vi "io_write_with_OPC_synchro.vi"(4 "Send *ESR? at the end (T)":bool=TRUE, 7 "Timeout in (0 = OPC timeout)":u32, 8 "error in":errorcluster, 10 "write buffer":string, 11 "VISA resource name":refnum<visa-resource-name>) -> (0 "error out":errorcluster, 3 "VISA resource name out":refnum<visa-resource-name>)   [LabVIEW 2014, in "rszvl_rsidr_core.lvlib"]
uses:
  rszvl_rsidr_core.lvlib
  type_Attribute.ctl
  type_Attribute_Data_Type.ctl
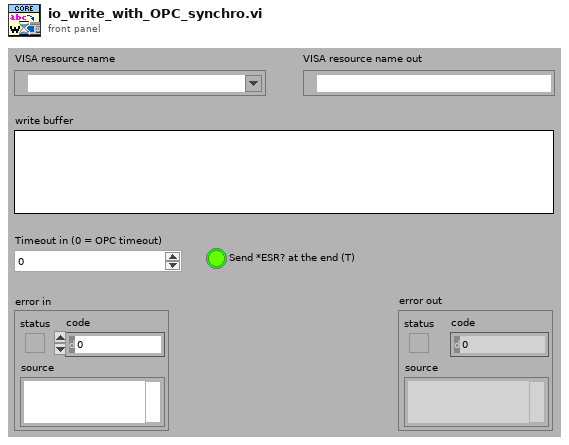
[diagram p1: front panel]
types:
  T1 = typedef "rszvl_rsidr_core.lvlib/type_Session_Data.ctl" = cluster{"Instr type":string, "Instr type for err. msg.":string, "Installed Options":string[], "OPC Timeout":i32, "Query Instrument Status":bool, "Check Range":bool, "Check Options":bool, "Add LF to Write":bool, "Simulate":bool, "Logging":bool, "Logging params":variant, "Interface Type":enum16{"Unknown", "GPIB", "VXI", "GPIB_VXI", "ASRL", "PXI", "TCPIP", "USB", "SOCKET"}, "Fast Sweep":i32, "AdditionalFlags":i32, "WaitBeforeWrite":i32, "WaitBeforeRead":i32, "BinDataChunkSize":i64}
  T2 = enum16{"Unknown", "GPIB", "VXI", "GPIB_VXI", "ASRL", "PXI", "TCPIP", "USB", "SOCKET"}
  T3 = typedef "rszvl_rsidr_core.lvlib/type_Attribute.ctl" = cluster{"Identifier":string, "Descriptive name":string, "Data Type":T4, "Command":string, "Access":u16, "Range Table":string, "Read Callback":string, "Write Callback":string, "Range Callback":string, "Check Callback":string, "Rngtable Callback":string, "Coerce Callback":string, "Supported Models":string, "Instrument Options":string, "Repeated Capabilities":string, "Check Status Callback":string, "Index":i32, "Flag: OPC Wait":bool, "Flag: Dont check status":bool, "Flag: Cache Only":bool}
  T4 = typedef "rszvl_rsidr_core.lvlib/type_Attribute_Data_Type.ctl" = enum16{"Integer 32", "Double", "String", "Boolean", "None", "Integer 64"}
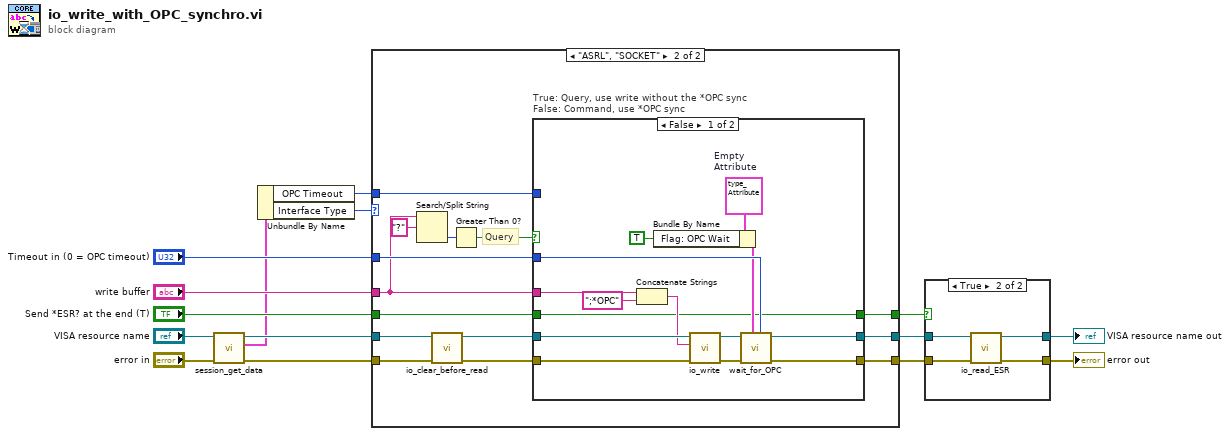
[diagram p0: block diagram]
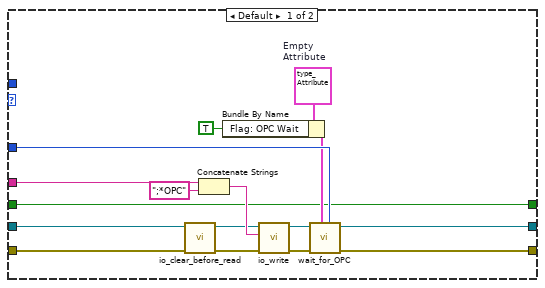
[diagram p3: hidden frame]
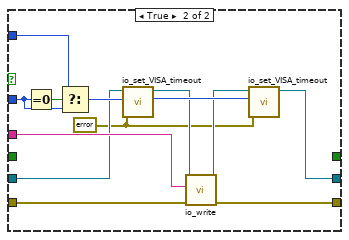
[diagram p4: hidden frame]
diagram:
  n1 = call "session_get_data.vi"("error in"="error in", "VISA resource name"="VISA resource name") -> ("error out"=w10:errorcluster, "Session User Data out"=w1:T1, "VISA resource name out"=w9:refnum<visa-resource-name>)  [unwired: 7 in]
  n2 = Unbundle By Name(w1) -> ("OPC Timeout"=w2:i32, "Interface Type"=w8:T2)
  n3 = case shown="\"ASRL\", \"SOCKET\"" w8 {
    tunnel: "Timeout in (0 = OPC timeout)" -> [w29 w45]
    tunnel: w10 -> [w28 w44]
    tunnel: w9 -> [w27 w43]
    tunnel: "write buffer" -> [w22 w37]
    tunnel: [w16 w36] -> w5
    tunnel: [w17 w35] -> w6
    tunnel: "Send *ESR? at the end (T)" -> [w18 w34]
    tunnel: [w18 w33] -> w7
    tunnel: w2 -> [_ w32]
    frame Default {
      w20 = T3 {"Identifier"="", "Descriptive name"="", "Data Type"=enum."Integer 32", "Command"="", "Access"=2, "Range Table"="", "Read Callback"="", "Write Callback"="", "Range Callback"="", "Check Callback"="", "Rngtable Callback"="", "Coerce Callback"="", "Supported Models"="", "Instrument Options"="", "Repeated Capabilities"="", "Check Status Callback"="", "Index"=0, "Flag: OPC Wait"=FALSE, "Flag: Dont check status"=FALSE, "Flag: Cache Only"=FALSE}  # Empty Attribute
      n4 = call "io_clear_before_read.vi"("error in"=w28, "VISA resource name"=w27) -> ("error out"=w26:errorcluster, "VISA resource name out"=w25:refnum<visa-resource-name>)  [unwired: 8 in]
      n5 = Concatenate Strings(w22, ";*OPC" ("string")) -> (w31:string)
      n6 = Bundle By Name(cluster=w20, "Flag: OPC Wait"=TRUE) -> (w19:T3)
      n7 = call "io_write.vi"("error in"=w26, "write buffer"=w31, "VISA resource name"=w25) -> ("error out"=w24:errorcluster, "VISA resource name out"=w23:refnum<visa-resource-name>)  [unwired: 7 in]
      n8 = call "wait_for_OPC.vi"("Timeout in (0 = OPC timeout)"=w29, "Attribute"=w19, "error in"=w24, "VISA resource name"=w23) -> ("error out"=w17:errorcluster, "VISA resource name out"=w16:refnum<visa-resource-name>)  [unwired: 6 in]
    }
    frame "ASRL", "SOCKET" {
      # "Query"
      n9 = Search/Split String(string=w37, search string/char (-)="?") -> (offset of match=w39:i32)  [unwired: 1 in, 2 out]
      n10 = call "io_clear_before_read.vi"("error in"=w44, "VISA resource name"=w43) -> ("error out"=w42:errorcluster, "VISA resource name out"=w41:refnum<visa-resource-name>)  [unwired: 8 in]
      n11 = Greater Than 0?(x=w39) -> (x > 0?=w38:bool)
      n12 = case "True: Query, use write without the *OPC sync\nFalse: Command, use *OPC sync" shown="False" w38 {
        tunnel: w37 -> [w51 w72]
        tunnel: w45 -> [w59 w70]
        tunnel: w42 -> [w58 w64]
        tunnel: w41 -> [w57 w67]
        tunnel: [w48 w62] -> w36
        tunnel: [w47 w63] -> w35
        tunnel: w34 -> [w46 _]
        tunnel: [w46 _] -> w33
        tunnel: w32 -> [_ w61]
        frame False {
          w53 = T3 {"Identifier"="", "Descriptive name"="", "Data Type"=enum."Integer 32", "Command"="", "Access"=2, "Range Table"="", "Read Callback"="", "Write Callback"="", "Range Callback"="", "Check Callback"="", "Rngtable Callback"="", "Coerce Callback"="", "Supported Models"="", "Instrument Options"="", "Repeated Capabilities"="", "Check Status Callback"="", "Index"=0, "Flag: OPC Wait"=FALSE, "Flag: Dont check status"=FALSE, "Flag: Cache Only"=FALSE}  # Empty Attribute
          n13 = Concatenate Strings(w51, ";*OPC" ("string")) -> (w49:string)
          n14 = Bundle By Name(cluster=w53, "Flag: OPC Wait"=TRUE) -> (w52:T3)
          n15 = call "io_write.vi"("error in"=w58, "write buffer"=w49, "VISA resource name"=w57) -> ("error out"=w56:errorcluster, "VISA resource name out"=w55:refnum<visa-resource-name>)  [unwired: 7 in]
          n16 = call "wait_for_OPC.vi"("Timeout in (0 = OPC timeout)"=w59, "Attribute"=w52, "error in"=w56, "VISA resource name"=w55) -> ("error out"=w47:errorcluster, "VISA resource name out"=w48:refnum<visa-resource-name>)  [unwired: 6 in]
        }
        frame True {
          w60 = errorcluster {"status"=FALSE, "code"=0, "source"=""} ("error in")
          n17 = Equal To 0?(x=w70) -> (x = 0?=w71:bool)
          n18 = Select(t=w61, s=w71, f=w70) -> (s? t:f=w69:u32)
          n19 = call "io_set_VISA_timeout.vi"("error in"=w60, "VISA Timeout"=w69, "VISA resource name"=w67) -> ("Old VISA Timeout"=w68:u32, "VISA resource name out"=w66:refnum<visa-resource-name>)  [unwired: 6 in, 1 out]
          n20 = call "io_write.vi"("error in"=w64, "write buffer"=w72, "VISA resource name"=w66) -> ("error out"=w63:errorcluster, "VISA resource name out"=w65:refnum<visa-resource-name>)  [unwired: 7 in]
          n21 = call "io_set_VISA_timeout.vi"("error in"=w60, "VISA Timeout"=w68, "VISA resource name"=w65) -> ("VISA resource name out"=w62:refnum<visa-resource-name>)  [unwired: 6 in, 2 out]
        }
      }
    }
  }
  n22 = case shown="True" w7 {
    tunnel: w6 -> [w74 w78]
    tunnel: w5 -> [w73 w77]
    tunnel: [w74 w76] -> w4
    tunnel: [w73 w75] -> w3
    frame False {
    }
    frame True {
      n23 = call "io_read_ESR.vi"("error in"=w78, "VISA resource name"=w77) -> ("error out"=w76:errorcluster, "VISA resource name out"=w75:refnum<visa-resource-name>)  [unwired: 7 in, 1 out]
    }
  }
  "VISA resource name out" <- w3
  "error out" <- w4
